vi "Asset Utilization.vi"(8 "error in (no error)":errorcluster, 11 "Logger in.lvclass":refnum<class "Logger.lvclass">) -> (0 "error out":errorcluster, 3 "Logger out.lvclass":refnum<class "Logger.lvclass">)   [LabVIEW 2024, in "Logger.lvclass"]
uses:
  Logger.lvclass
  Logger.lvclass/Logger.ctl
panel:
  out "Logging":bool
  out "Status":string
  out "utilizationIdentifier":string
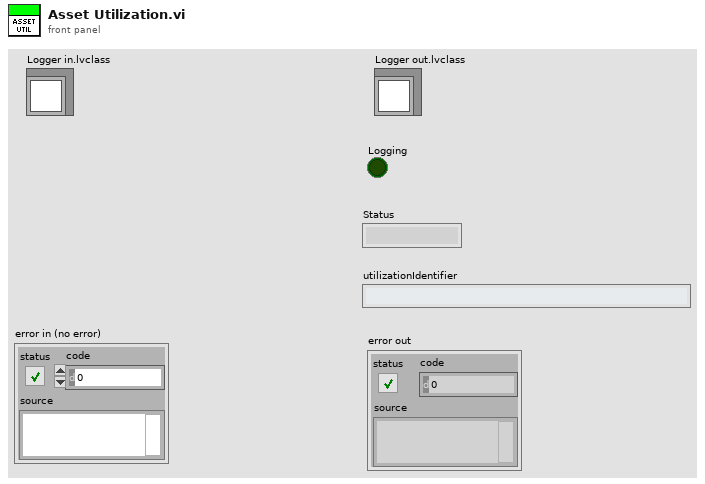
[diagram p1: front panel]
types:
  T1 = cluster{"modelName":string, "modelNumber":i32, "serialNumber":string, "vendorName":string, "busType":string}
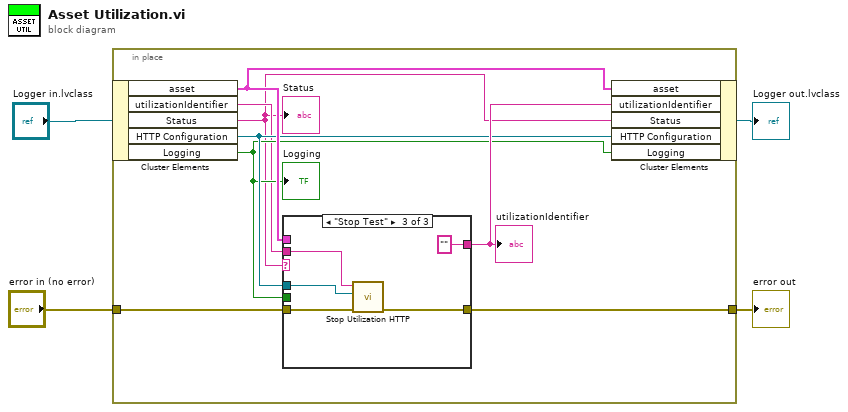
[diagram p0: block diagram]
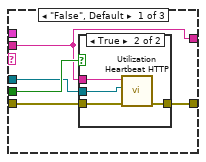
[diagram p2: hidden frame]
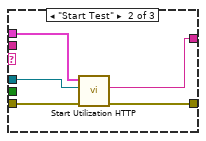
[diagram p4: hidden frame]
diagram:
  n1 = in-place {
    in-place-border: "error in (no error)" -> [w10]
    in-place-border: [w12] -> w1
    n2 = in-place-cluster #1("Logger in.lvclass") -> ("asset"=w11:T1, "utilizationIdentifier"=w6:string, "Status"=w5:string, "HTTP Configuration"=w8:refnum<class "NI Skyline Configuration HTTP.lvclass">, "Logging"=w7:bool)
    "Status" <- w5
    "Logging" <- w7
    n3 = case shown="\"Stop Test\"" w5 {
      tunnel: [w13 w27 w29] -> w12
      tunnel: [w15 w26 "" ("utilizationIdentifier")] -> w9
      tunnel: w11 -> [_ w25 _]
      tunnel: w8 -> [w16 w23 w31]
      tunnel: w10 -> [w14 w24 w30]
      tunnel: w6 -> [w15 _ w32]
      tunnel: w7 -> [w17 _ _]
      frame "False", Default {
        n4 = case shown="True" w17 {
          tunnel: w16 -> [_ w22]
          tunnel: w15 -> [_ w21]
          tunnel: w14 -> [w18 w20]
          tunnel: [w18 w19] -> w13
          frame False {
          }
          frame True {
            n5 = call "Utilization Heartbeat HTTP.vi"("error in (no error)"=w20, "configuration"=w22, "utilizationIdentifier"=w21) -> ("error out"=w19:errorcluster)  [unwired: 8 in]
          }
        }
      }
      frame "Start Test" {
        n6 = call "Start Utilization HTTP.vi"("error in (no error)"=w24, "configuration"=w23, "asset"=w25) -> ("error out"=w27:errorcluster, "utilizationIdentifier"=w26:string)  [unwired: 6 in, 1 out]
      }
      frame "Stop Test" {
        n7 = call "Stop Utilization HTTP.vi"("error in (no error)"=w30, "configuration"=w31, "utilizationIdentifier"=w32) -> ("error out"=w29:errorcluster)  [unwired: 8 in]
      }
    }
    "utilizationIdentifier" <- w9
    n8 = in-place-cluster #1("asset"=w11, "utilizationIdentifier"=w9, "Status"=w5, "HTTP Configuration"=w8, "Logging"=w7) -> (→"Logger out.lvclass":refnum<class "Logger.lvclass">)
  }
  "error out" <- w1
